vi "2100_IVIO_KGD.vi"(0 "Semiconductor Module Context":T6, 1 "All_Scripts":string[][](array[string]), 2 "Master_Register_Data_Array_In":T1 {"Address" format="%.0x"}, 3 "Publishable IDs":string[](array[string])=["LowPower", "Active"], 4 "USID":T3 max=15, 5 "Error In":errorcluster, 6 "aperture time":dbl=0.001, 7 "SMU_Pins":string[](array[string])=["VSU"], 8 "Meas_Delay":dbl format="%#_13g", 10 "Low Power_SMU_Settings":T5={"Level"=1.8, "Level Range"=6.0, "Limit"=0.001, "Limit Range"=0.001, "Sense"=1009} {"Limit" format="%#_6p"; "Limit Range" format="%#_6p"; "Sense" items=["Local"=1008, "Remote"=1009]}, 11 "HSDIO_Pins":string[](array[string])=["CLK", "SDA"], 12 "Active_SMU_Settings":T5={"Level"=1.8, "Level Range"=6.0, "Limit"=0.01, "Limit Range"=0.01, "Sense"=1009} {"Limit" format="%#_6p"; "Limit Range" format="%#_6p"; "Sense" items=["Local"=1008, "Remote"=1009]}, 13 "Script Name":string="IVIOKGD") -> (15 "Master_Register_Data_Array_Out":T1 {"Address" format="%.0x"}, 19 "Error Out":errorcluster)   [LabVIEW 2013]
uses:
  Controls/USID.ctl
  <vilib>/NI_TestStand_SemiconductorModule/NI_TestStand_Semiconductor_Module.lvlibp/PinMap/General/SemiconductorModuleContext.ctl
  <instrlib>/niDCPower/nidcpower.llb/niDCPower Sense.ctl
  Controls/Master_Reg_Data_Array.ctl
  Controls/Reg_Address_Data.ctl
  <vilib>/NI_TestStand_SemiconductorModule/NI_TestStand_Semiconductor_Module.lvlibp/PinMap/DC Power/PinsToNIDCPowerSessions.vi
  <vilib>/NI_TestStand_SemiconductorModule/NI_TestStand_Semiconductor_Module.lvlibp/PinMap/General/Publish/PublishDataDouble2D.vi
  <vilib>/NI_TestStand_SemiconductorModule/NI_TestStand_Semiconductor_Module.lvlibp/PinMap/PinQueryContext/MultiplePinMultipleSessionQueryContext/MultiplePinMultipleSessionQueryContext.lvclass
  <vilib>/NI_TestStand_SemiconductorModule/NI_TestStand_Semiconductor_Module.lvlibp
panel:
  in  "Tab Control":enum32{"Test Info", "Instrument Settings"}(tab)
  out "current measurements":dbl[][](array[numeric])
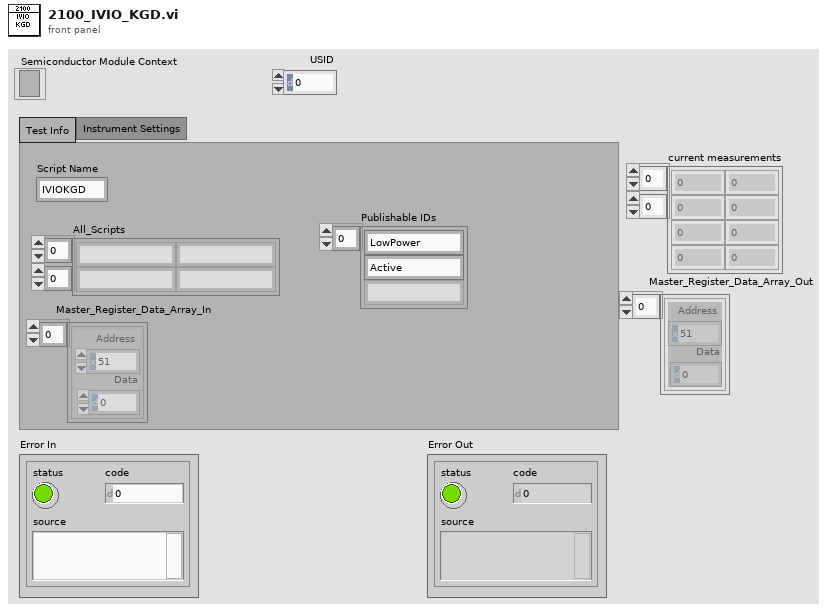
[diagram p1: front panel]
types:
  T1 = typedef "Master_Reg_Data_Array.ctl" = T2[]
  T2 = typedef "Reg_Address_Data.ctl" = cluster{"Address":u8, "Data":u8}
  T3 = typedef "USID.ctl" = u8
  T4 = typedef "niDCPower Sense.ctl" = i32
  T5 = cluster{"Level":dbl, "Level Range":dbl, "Limit":dbl, "Limit Range":dbl, "Sense":T4}
  T6 = typedef "NI_TestStand_Semiconductor_Module.lvlibp/SemiconductorModuleContext.ctl" = refnum<k7>
  T7 = typedef "Script Functions_Array.ctl" = enum16{"Reg_Write", "Bit_Write", "Delay", "Read", "Measure"}[]
  T8 = enum16{"Reg_Write", "Bit_Write", "Delay", "Read"}
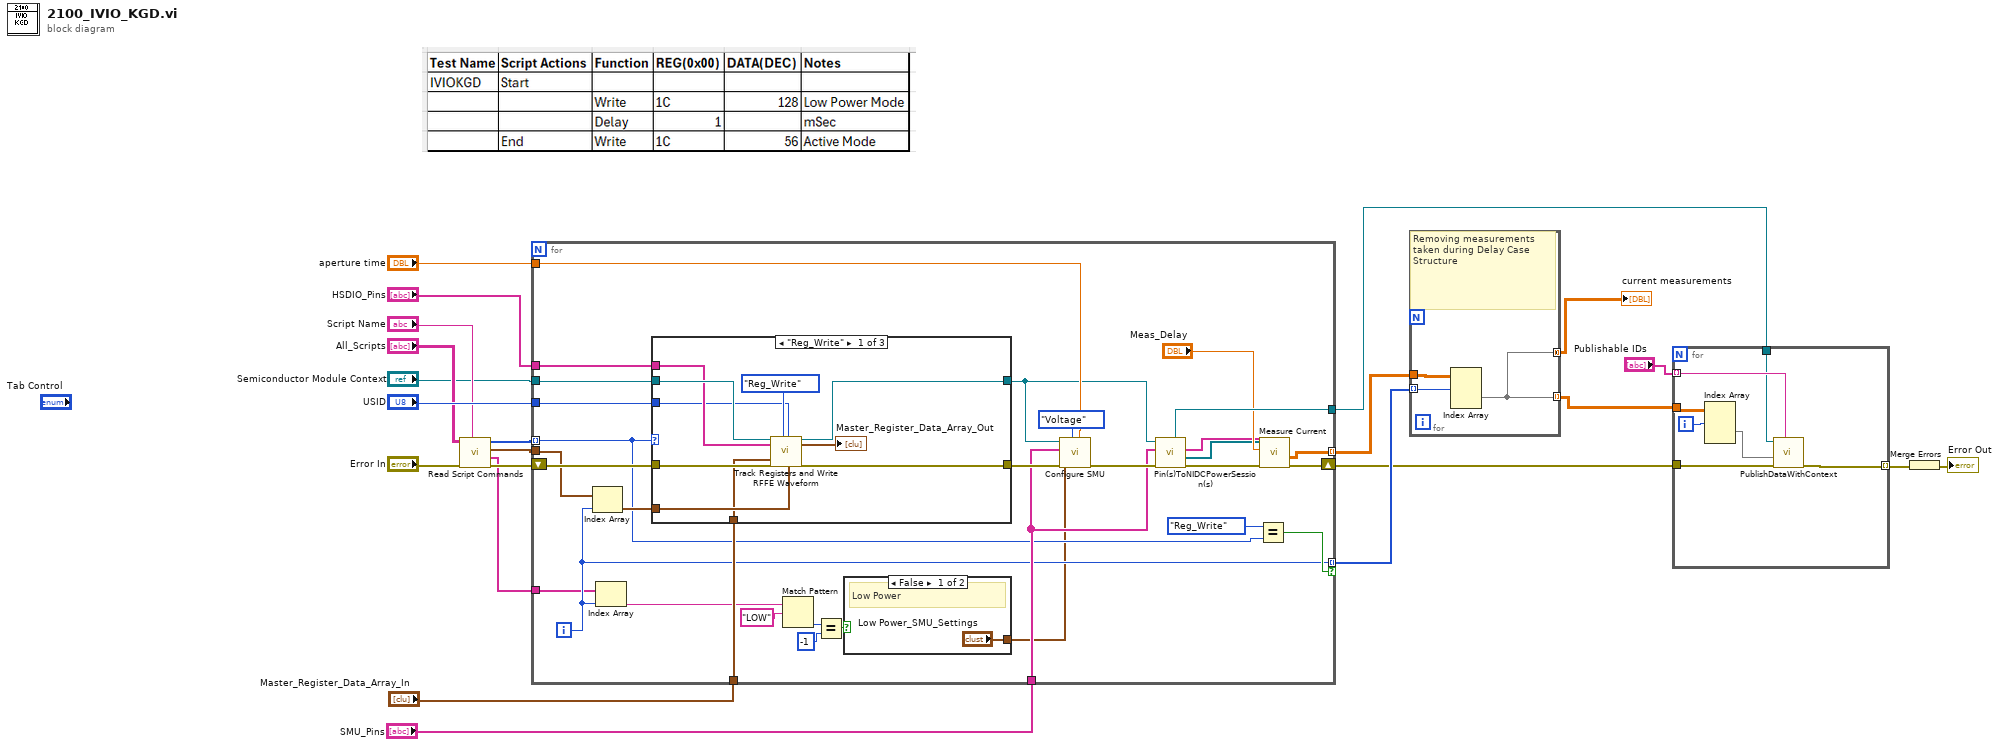
[diagram p0: block diagram]
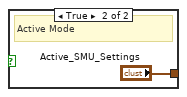
[diagram p2: hidden frame]
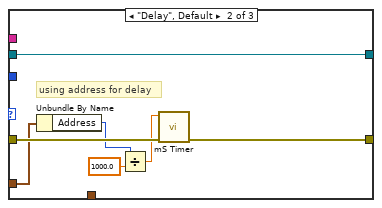
[diagram p3: hidden frame]
diagram:
  n1 = call "Read Script Commands.vi"("Test Name"="Script Name", "Error In"="Error In", "All_Scripts"="All_Scripts") -> ("Error Out"=w17:errorcluster, "Script_Note"=w1:string[], "Script_Data"=w18:T2[], "Script_Functions"=w19:T7)  [unwired: 5 in]
  n2 = for {
    tunnel: "USID" -> [w39]
    tunnel: w19 -> [w32] mode=indexing
    tunnel: w18 -> [w50]
    tunnel: "Semiconductor Module Context" -> [w52]
    tunnel: "HSDIO_Pins" -> [w51]
    tunnel: "aperture time" -> [w47]
    tunnel: "SMU_Pins" -> [w43]
    tunnel: [w42] -> w9 mode=indexing
    shift-right: [w41] -> w6
    shift-left: w17 -> [w53]
    tunnel: "Master_Register_Data_Array_In" -> [w40]
    tunnel: [w38] -> w5
    tunnel: [w26] -> w8 mode=indexing if=w31
    tunnel: w1 -> [w25]
    i -> [w26]
    n3 = Index Array(array=w50, index=w26) -> (element=w49:T2)
    n4 = Index Array(array=w25, index=w26) -> (element=w24:string)
    n5 = case shown="\"Reg_Write\"" w32 {
      tunnel: w49 -> [w59 w71 _]
      tunnel: w53 -> [w65 w72 w74]
      tunnel: w39 -> [w56 _ _]
      tunnel: w52 -> [w63 w69 w73]
      tunnel: w51 -> [w61 _ _]
      tunnel: [w64 w70 w74] -> w48
      tunnel: [w62 w69 w73] -> w44
      tunnel: w40 -> [w58 _ _]
      frame "Reg_Write" {
        n6 = call "Track Registers and Write RFFE Waveform.vi"("Semiconductor Module Context"=w63, "Pins"=w61, "Master_Register_Data_Array_In"=w58, "Error In"=w65, "Script_Functions"=enum16{"Reg_Write", "Bit_Write"}."Reg_Write", "USID"=w56, "Reg_Address_Data"=w59) -> ("Semiconductor Module Context Out"=w62:T6, "Master_Register_Data_Array_Out"=→"Master_Register_Data_Array_Out":T1, "Error Out"=w64:errorcluster)  [unwired: 10 in]
      }
      frame "Delay", Default {
        # "using address for delay"
        n7 = Unbundle By Name(w71) -> ("Address"=w67:u8)
        n8 = Divide(x=w67, y=1000.0) -> (x/y=w66:dbl)
        n9 = call "mS Timer.vi"("Error In"=w72, "Delay(S)"=w66) -> ("Error Out"=w70:errorcluster)  [unwired: 9 in]
      }
      frame "Read" {
      }
    }
    n10 = Match Pattern(string=w24, regular expression="LOW") -> (offset past match=w28:i32)  [unwired: 1 in, 3 out]
    n11 = Equal?(x=w28, y=-1) -> (x = y?=w30:bool)
    n12 = case shown="False" w30 {
      tunnel: ["Low Power_SMU_Settings" "Active_SMU_Settings"] -> w23
      frame False {
        # "Low Power"
      }
      frame True {
        # "Active Mode"
      }
    }
    n13 = call "Configure SMU.vi"("aperture time"=w47, "Source Mode"=enum16{"Voltage", "Current"}."Voltage", "error in (no error)"=w48, "Settings"=w23, "Pins"=w43, "Semiconductor Module Context"=w44) -> ("error out"=w45:errorcluster)  [unwired: 5 in]
    n14 = call-poly <vilib>:"Pin(s)ToNIDCPowerSession(s).vi"("error in (no error)"=w45, "Pins"=w43, "Semiconductor Module Context"=w44) -> ("error out"=w36:errorcluster, "Instrument Sessions"=w34:refnum<k15>[], "Channel Lists"=w35:string[], "Pin Query Context"=w38:refnum<class "MultiplePinMultipleSessionQueryContext.lvclass">)  [unwired: 4 in, 1 out]
    n15 = Equal?(x=T8."Reg_Write" ("Enum"), y=w32) -> (x = y?=w31:bool)
    n16 = call "Measure Current.vi"("Channel Lists"=w35, "error in (no error)"=w36, "Delay Time (s)"="Meas_Delay", "DCPower Sessions In"=w34) -> ("error out"=w41:errorcluster, "current measurements"=w42:dbl[][])  [unwired: 5 in, 1 out]
  }
  n17 = for {
    tunnel: w9 -> [w77]
    tunnel: w8 -> [w76] mode=indexing
    tunnel: [w75] -> w4 mode=indexing
    tunnel: [w75] -> w7 mode=concatenating
    # "Removing measurements taken during Delay Case Structure"
    n18 = Index Array(array=w77, index (dim 0)=w76) -> (element=w75:dbl[][])  [unwired: 2 in]
  }
  "current measurements" <- w7
  n19 = for {
    tunnel: "Publishable IDs" -> [w84] mode=indexing
    tunnel: [w83] -> w11 mode=indexing
    tunnel: w6 -> [w82]
    tunnel: w5 -> [w81]
    tunnel: w4 -> [w80]
    i -> [w79]
    n20 = Index Array(array=w80, index (dim 0)=w79) -> (element=w78:dbl[][])  [unwired: 2 in]
    n21 = call-poly <vilib>:"PublishDataWithContext.vi"("Published Data Id"=w84, "error in (no error)"=w82, "Data In"=w78, "Pin Query Context"=w81) -> ("error out"=w83:errorcluster)  [unwired: 6 in, 1 out]
  }
  n22 = Merge Errors(w11) -> (→"Error Out":errorcluster)
